vi "After Launch Init.vi"(8 "error in (no error)":errorcluster, 11 "CS++Fgen in":refnum<class "CS++Fgen.lvclass">) -> (0 "error out":errorcluster, 3 "CS++Fgen out":refnum<class "CS++Fgen.lvclass">)   [LabVIEW 2013, in "CS++Fgen.lvlib" / "CS++Fgen.lvclass"]
doc: "Use <b>Pre Launch init.vi</b> method for sanity checks that are supposed to prevent the actor from launching if they fail. Use <B>this</B> method instead to initialize this actor when it has been activated. A corresponding high priority message will become dispatched before the <B>Actor Core.vi</b> is called.\n\n<b>Derived classed should call the parent methode first</b> and their own initialization code after.\n\nRefer also to the ongoing discussion at https://decibel.ni.com/content/message/57394#57394."
uses:
  CS++Fgen.lvclass
  Core/Classes/CS++ProcessVariables/ProcessVariable/PV.lvclass
  Core/Classes/CS++ProcessVariables/SVConnection/SVConnection.lvclass
  CS++Fgen.lvclass/CS++Fgen.ctl
  Core/Classes/CS++ProcessVariables/ProcessVariable/PV.lvclass/PV.ctl
  Core/Classes/CS++ProcessVariables/PVConnection/PVConnection.lvclass/PVConnection.ctl
  Core/Actors/CS++DeviceActor/CS++DeviceActor.lvclass
  Core/Actors/CS++DeviceActor/CS++DeviceActor.lvclass/CS++DeviceActor.ctl
  <vilib>/ActorFramework/Actor/Actor.lvclass/Actor.ctl
  <vilib>/ActorFramework/Message Enqueuer/Message Enqueuer.lvclass/Message Enqueuer.ctl
  CS++DCPwr Messages/Measure [MSR] Msg/Measure [MSR] Msg.lvclass/Measure [MSR] Msg.ctl
  CS++DCPwr Messages/Measure [MSR] Msg/Write channel name.vi
  CS++DCPwr Messages/Measure [MSR] Msg/Write measurement type.vi
  Core/Classes/CS++ProcessVariables/ProcessVariable/Write PV URL.vi
  Core/Classes/CS++ProcessVariables/ProcessVariable/Write Data.vi
  Core/Classes/CS++ProcessVariables/ProcessVariable/Write Error.vi
  Core/Classes/CS++ProcessVariables/ProcessVariable/Write Quality.vi
  Core/Classes/CS++ProcessVariables/ProcessVariable/Write status.vi
  Core/Classes/CS++ProcessVariables/ProcessVariable/Write Timestamp.vi
  Core/Classes/CS++ProcessVariables/PVConnection/Write PV URL.vi
  <vilib>/ActorFramework/Message Enqueuer/Init from Existing Queue.vi
  <vilib>/ActorFramework/Message Enqueuer/Message Enqueuer.lvclass
  CS++DCPwr Messages/Measure [MSR] Msg/Measure [MSR] Msg.lvclass
  <vilib>/ActorFramework/Actor/Actor.lvclass
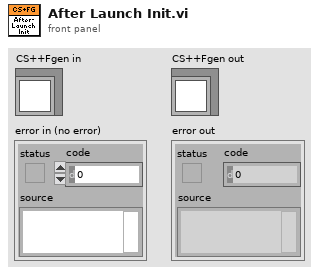
[diagram p1: front panel]
types:
  T1 = cluster{"Write Access":enum8{"Allowed", "Required", "None"}, "Read Access":enum8{"Allowed", "Required", "None"}}
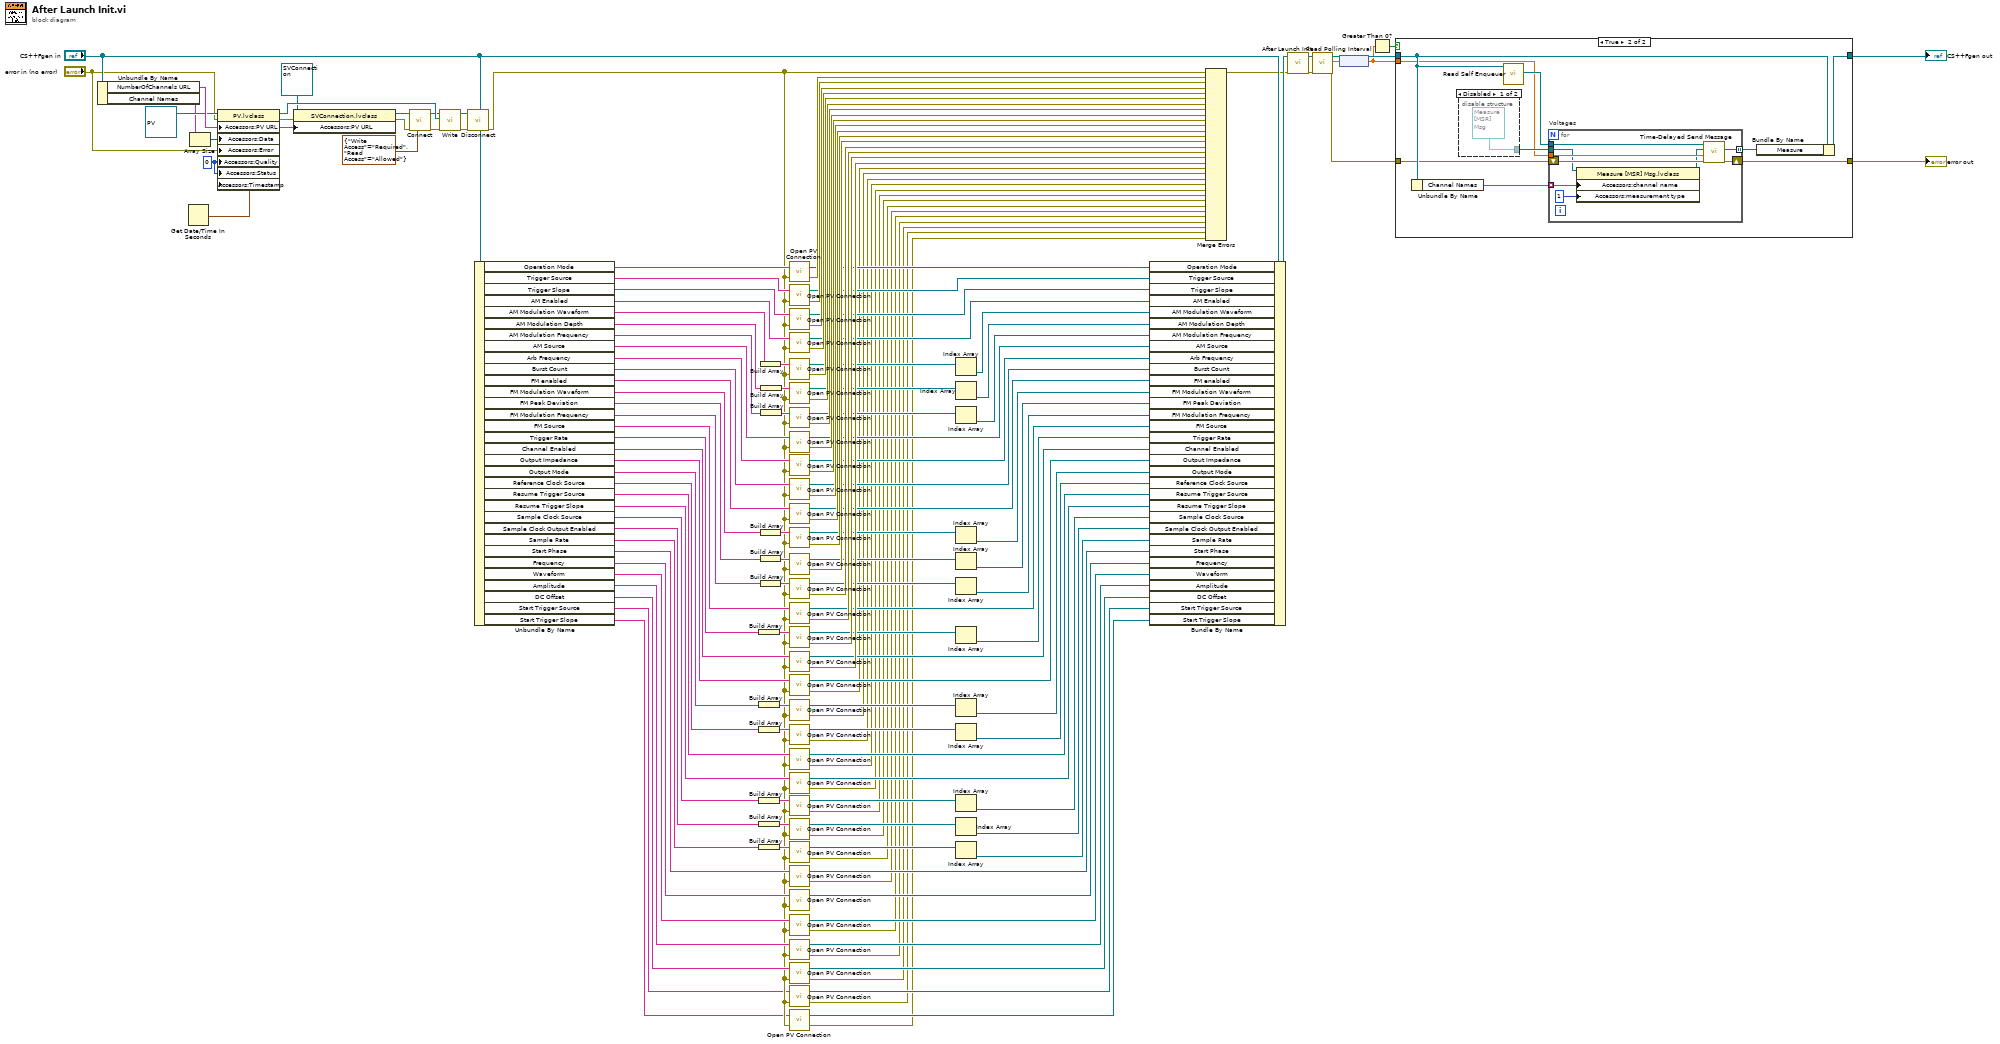
[diagram p0: block diagram]
diagram:
  w137 = 0 ("Quality")
  n1 = Unbundle By Name("CS++Fgen in") -> ("NumberOfChannels URL"=w141:string, "Channel Names"=w134:string[])
  n2 = Get Date/Time In Seconds() -> (seconds since 1Jan1904=w138:timestamp)
  n3 = Array Size(array=w134) -> (size(s)=w136:i32)
  n4 = property class="PV.lvclass"(reference=refnum<class "PV.lvclass"> refnum ("CS++ProcessVariables.lvlib:PV.lvclass"), error in="error in (no error)", "Accessors:PV URL"=w141, "Accessors:Data"=w136, "Accessors:Error"="error in (no error)", "Accessors:Quality"=w137, "Accessors:Status"=w137, "Accessors:Timestamp"=w138) -> (reference out=w147:refnum<class "PV.lvclass">, error out=w142:errorcluster)
  n5 = property class="SVConnection.lvclass"(reference=refnum<class "SVConnection.lvclass"> refnum ("CS++ProcessVariables.lvlib:SVConnection.lvclass"), error in=w142, "Accessors:PV URL"=w141) -> (reference out=w140:refnum<class "SVConnection.lvclass">, error out=w143:errorcluster)
  n6 = call-dynamic "Connect.vi"("Access"=T1 {"Write Access"=enum."Required", "Read Access"=enum."Allowed"}, "error in (no error)"=w143, "PVConnection in"=w140) -> ("error out"=w146:errorcluster, "PVConnection out"=w145:refnum<class "SVConnection.lvclass">)  [unwired: 7 in]
  n7 = call-dynamic "Write.vi"("error in (no error)"=w146, "PV"=w147, "PVConnection in"=w145) -> ("error out"=w149:errorcluster, "PVConnection out"=w148:refnum<class "SVConnection.lvclass">)  [unwired: 7 in]
  n8 = call-dynamic "Disconnect.vi"("error in (no error)"=w149, "PVConnection in"=w148) -> ("error out"=w7:errorcluster)  [unwired: 8 in, 1 out]
  n9 = Unbundle By Name("CS++Fgen in") -> ("Operation Mode"=w133:string[], "Trigger Source"=w101:string[], "Trigger Slope"=w100:string[], "AM Enabled"=w97:string[], "AM Modulation Waveform"=w95:string, "AM Modulation Depth"=w91:string, "AM Modulation Frequency"=w90:string, "AM Source"=w83:string[], "Arb Frequency"=w81:string[], "Burst Count"=w79:string[], "FM enabled"=w77:string[], "FM Modulation Waveform"=w75:string, "FM Peak Deviation"=w71:string, "FM Modulation Frequency"=w70:string, "FM Source"=w69:string[], "Trigger Rate"=w61:string, "Channel Enabled"=w57:string[], "Output Impedance"=w55:string[], "Output Mode"=w50:string, "Reference Clock Source"=w45:string, "Resume Trigger Source"=w42:string[], "Resume Trigger Slope"=w41:string[], "Sample Clock Source"=w34:string, "Sample Clock Output Enabled"=w29:string, "Sample Rate"=w24:string, "Start Phase"=w21:string[], "Frequency"=w20:string[], "Waveform"=w19:string[], "Amplitude"=w18:string[], "DC Offset"=w17:string[], "Start Trigger Source"=w6:string[], "Start Trigger Slope"=w5:string[])
  n10 = Build Array(w61) -> (w60:string[])
  n11 = Build Array(w50) -> (w51:string[])
  n12 = Build Array(w45) -> (w47:string[])
  n13 = Build Array(w34) -> (w35:string[])
  n14 = Build Array(w29) -> (w31:string[])
  n15 = Build Array(w24) -> (w25:string[])
  n16 = Build Array(w95) -> (w94:string[])
  n17 = Build Array(w75) -> (w74:string[])
  n18 = Build Array(w71) -> (w68:string[])
  n19 = Build Array(w70) -> (w67:string[])
  n20 = Build Array(w91) -> (w93:string[])
  n21 = Build Array(w90) -> (w92:string[])
  n22 = call "Open PV Connection.vi"("Error In"=w7, "URLs"=w133) -> ("Error Out"=w132:errorcluster, "PV Connections"=w113:refnum<class "SVConnection.lvclass">[])
  n23 = call "Open PV Connection.vi"("Error In"=w7, "URLs"=w101) -> ("Error Out"=w131:errorcluster, "PV Connections"=w99:refnum<class "SVConnection.lvclass">[])
  n24 = call "Open PV Connection.vi"("Error In"=w7, "URLs"=w100) -> ("Error Out"=w130:errorcluster, "PV Connections"=w98:refnum<class "SVConnection.lvclass">[])
  n25 = call "Open PV Connection.vi"("Error In"=w7, "URLs"=w97) -> ("Error Out"=w129:errorcluster, "PV Connections"=w96:refnum<class "SVConnection.lvclass">[])
  n26 = call "Open PV Connection.vi"("Error In"=w7, "URLs"=w94) -> ("Error Out"=w128:errorcluster, "PV Connections"=w89:refnum<class "SVConnection.lvclass">[])
  n27 = call "Open PV Connection.vi"("Error In"=w7, "URLs"=w93) -> ("Error Out"=w127:errorcluster, "PV Connections"=w87:refnum<class "SVConnection.lvclass">[])
  n28 = call "Open PV Connection.vi"("Error In"=w7, "URLs"=w92) -> ("Error Out"=w126:errorcluster, "PV Connections"=w84:refnum<class "SVConnection.lvclass">[])
  n29 = call "Open PV Connection.vi"("Error In"=w7, "URLs"=w83) -> ("Error Out"=w125:errorcluster, "PV Connections"=w82:refnum<class "SVConnection.lvclass">[])
  n30 = call "Open PV Connection.vi"("Error In"=w7, "URLs"=w81) -> ("Error Out"=w124:errorcluster, "PV Connections"=w80:refnum<class "SVConnection.lvclass">[])
  n31 = call "Open PV Connection.vi"("Error In"=w7, "URLs"=w79) -> ("Error Out"=w123:errorcluster, "PV Connections"=w78:refnum<class "SVConnection.lvclass">[])
  n32 = call "Open PV Connection.vi"("Error In"=w7, "URLs"=w77) -> ("Error Out"=w122:errorcluster, "PV Connections"=w76:refnum<class "SVConnection.lvclass">[])
  n33 = call "Open PV Connection.vi"("Error In"=w7, "URLs"=w74) -> ("Error Out"=w121:errorcluster, "PV Connections"=w73:refnum<class "SVConnection.lvclass">[])
  n34 = call "Open PV Connection.vi"("Error In"=w7, "URLs"=w68) -> ("Error Out"=w120:errorcluster, "PV Connections"=w66:refnum<class "SVConnection.lvclass">[])
  n35 = call "Open PV Connection.vi"("Error In"=w7, "URLs"=w67) -> ("Error Out"=w119:errorcluster, "PV Connections"=w65:refnum<class "SVConnection.lvclass">[])
  n36 = call "Open PV Connection.vi"("Error In"=w7, "URLs"=w69) -> ("Error Out"=w118:errorcluster, "PV Connections"=w62:refnum<class "SVConnection.lvclass">[])
  n37 = call "Open PV Connection.vi"("Error In"=w7, "URLs"=w60) -> ("Error Out"=w117:errorcluster, "PV Connections"=w59:refnum<class "SVConnection.lvclass">[])
  n38 = call "Open PV Connection.vi"("Error In"=w7, "URLs"=w57) -> ("Error Out"=w116:errorcluster, "PV Connections"=w56:refnum<class "SVConnection.lvclass">[])
  n39 = call "Open PV Connection.vi"("Error In"=w7, "URLs"=w55) -> ("Error Out"=w53:errorcluster, "PV Connections"=w54:refnum<class "SVConnection.lvclass">[])
  n40 = call "Open PV Connection.vi"("Error In"=w7, "URLs"=w51) -> ("Error Out"=w48:errorcluster, "PV Connections"=w52:refnum<class "SVConnection.lvclass">[])
  n41 = call "Open PV Connection.vi"("Error In"=w7, "URLs"=w47) -> ("Error Out"=w43:errorcluster, "PV Connections"=w46:refnum<class "SVConnection.lvclass">[])
  n42 = call "Open PV Connection.vi"("Error In"=w7, "URLs"=w42) -> ("Error Out"=w38:errorcluster, "PV Connections"=w40:refnum<class "SVConnection.lvclass">[])
  n43 = call "Open PV Connection.vi"("Error In"=w7, "URLs"=w41) -> ("Error Out"=w37:errorcluster, "PV Connections"=w39:refnum<class "SVConnection.lvclass">[])
  n44 = call "Open PV Connection.vi"("Error In"=w7, "URLs"=w35) -> ("Error Out"=w32:errorcluster, "PV Connections"=w36:refnum<class "SVConnection.lvclass">[])
  n45 = call "Open PV Connection.vi"("Error In"=w7, "URLs"=w31) -> ("Error Out"=w27:errorcluster, "PV Connections"=w30:refnum<class "SVConnection.lvclass">[])
  n46 = call "Open PV Connection.vi"("Error In"=w7, "URLs"=w25) -> ("Error Out"=w22:errorcluster, "PV Connections"=w26:refnum<class "SVConnection.lvclass">[])
  n47 = call "Open PV Connection.vi"("Error In"=w7, "URLs"=w21) -> ("Error Out"=w11:errorcluster, "PV Connections"=w16:refnum<class "SVConnection.lvclass">[])
  n48 = call "Open PV Connection.vi"("Error In"=w7, "URLs"=w20) -> ("PV Connections"=w15:refnum<class "SVConnection.lvclass">[])  [unwired: 1 out]
  n49 = call "Open PV Connection.vi"("Error In"=w7, "URLs"=w19) -> ("Error Out"=w10:errorcluster, "PV Connections"=w14:refnum<class "SVConnection.lvclass">[])
  n50 = call "Open PV Connection.vi"("Error In"=w7, "URLs"=w18) -> ("Error Out"=w9:errorcluster, "PV Connections"=w13:refnum<class "SVConnection.lvclass">[])
  n51 = call "Open PV Connection.vi"("Error In"=w7, "URLs"=w17) -> ("Error Out"=w8:errorcluster, "PV Connections"=w12:refnum<class "SVConnection.lvclass">[])
  n52 = call "Open PV Connection.vi"("Error In"=w7, "URLs"=w6) -> ("Error Out"=w2:errorcluster, "PV Connections"=w4:refnum<class "SVConnection.lvclass">[])
  n53 = call "Open PV Connection.vi"("Error In"=w7, "URLs"=w5) -> ("Error Out"=w1:errorcluster, "PV Connections"=w3:refnum<class "SVConnection.lvclass">[])
  n54 = Index Array(array=w89) -> (element=w88:refnum<class "SVConnection.lvclass">)  [unwired: 1 in]
  n55 = Index Array(array=w87) -> (element=w86:refnum<class "SVConnection.lvclass">)  [unwired: 1 in]
  n56 = Index Array(array=w84) -> (element=w85:refnum<class "SVConnection.lvclass">)  [unwired: 1 in]
  n57 = Index Array(array=w73) -> (element=w72:refnum<class "SVConnection.lvclass">)  [unwired: 1 in]
  n58 = Index Array(array=w66) -> (element=w64:refnum<class "SVConnection.lvclass">)  [unwired: 1 in]
  n59 = Index Array(array=w65) -> (element=w63:refnum<class "SVConnection.lvclass">)  [unwired: 1 in]
  n60 = Index Array(array=w59) -> (element=w58:refnum<class "SVConnection.lvclass">)  [unwired: 1 in]
  n61 = Index Array(array=w52) -> (element=w49:refnum<class "SVConnection.lvclass">)  [unwired: 1 in]
  n62 = Index Array(array=w46) -> (element=w44:refnum<class "SVConnection.lvclass">)  [unwired: 1 in]
  n63 = Index Array(array=w36) -> (element=w33:refnum<class "SVConnection.lvclass">)  [unwired: 1 in]
  n64 = Index Array(array=w30) -> (element=w28:refnum<class "SVConnection.lvclass">)  [unwired: 1 in]
  n65 = Index Array(array=w26) -> (element=w23:refnum<class "SVConnection.lvclass">)  [unwired: 1 in]
  n66 = Bundle By Name(cluster="CS++Fgen in", "Operation Mode"=w113, "Trigger Source"=w99, "Trigger Slope"=w98, "AM Enabled"=w96, "AM Modulation Waveform"=w88, "AM Modulation Depth"=w86, "AM Modulation Frequency"=w85, "AM Source"=w82, "Arb Frequency"=w80, "Burst Count"=w78, "FM enabled"=w76, "FM Modulation Waveform"=w72, "FM Peak Deviation"=w64, "FM Modulation Frequency"=w63, "FM Source"=w62, "Trigger Rate"=w58, "Channel Enabled"=w56, "Output Impedance"=w54, "Output Mode"=w49, "Reference Clock Source"=w44, "Resume Trigger Source"=w40, "Resume Trigger Slope"=w39, "Sample Clock Source"=w33, "Sample Clock Output Enabled"=w28, "Sample Rate"=w23, "Start Phase"=w16, "Frequency"=w15, "Waveform"=w14, "Amplitude"=w13, "DC Offset"=w12, "Start Trigger Source"=w4, "Start Trigger Slope"=w3) -> (w114:refnum<class "CS++Fgen.lvclass">)
  n67 = Merge Errors(w7, w132, w131, w130, w129, w128, w127, w126, w125, w124, w123, w122, w121, w120, w119, w118, w117, w116, w53, w48, w43, w38, w37, w32, w27, w22, w11, w10, w9, w8, w2, w1) -> (w102:errorcluster)
  n68 = call-parent "After Launch Init.vi"("error in (no error)"=w102, "CS++DeviceActor in"=w114) -> ("error out"=w105:errorcluster, "CS++DeviceActor out"=w106:refnum<class "CS++Fgen.lvclass">)  [unwired: 8 in]
  n69 = call "Read Polling Interval.vi"("error in (no error)"=w105, "CS++DeviceActor in"=w106) -> ("error out"=w110:errorcluster, "Polling Interval"=w109:dbl[unit], "CS++DeviceActor out"=w111:refnum<class "CS++Fgen.lvclass">)  [unwired: 7 in]
  n70 = node(w109) -> (w108:dbl)
  n71 = Greater Than 0?(x=w108) -> (x > 0?=w107:bool)
  n72 = case shown="True" w107 {
    tunnel: [w151 w160] -> w104
    tunnel: [w150 w152] -> w103
    tunnel: w111 -> [w151 w159]
    tunnel: w110 -> [w150 w156]
    tunnel: w108 -> [_ w155]
    frame False {
    }
    frame True {
      n73 = Unbundle By Name(w159) -> ("Channel Names"=w154:string[])
      n74 = disable-structure shown="Disabled" {
        disable-tunnel: [refnum<class "Measure [MSR] Msg.lvclass"> refnum ("CS++DCPwr.lvlib:Measure [MSR] Msg.lvclass") _] -> w158
        frame Disabled {
        }
        frame Enabled {
        }
      }
      n75 = call <vilib>:"Read Self Enqueuer.vi"("Actor"=w159) -> ("Self Enqueuer"=w157:refnum<class "Message Enqueuer.lvclass">)  [unwired: 10 in]
      n76 = for "Voltages" {
        tunnel: w157 -> [w169]
        tunnel: w155 -> [w167]
        tunnel: [w166] -> w153 mode=indexing
        tunnel: w158 -> [w162]
        shift-right: [w170] -> w152
        shift-left: w156 -> [w168]
        tunnel: w154 -> [w165] mode=indexing
        n77 = property class="Measure [MSR] Msg.lvclass"(reference=w162, "Accessors:channel name"=w165, "Accessors:measurement type"=1 ("measurement type (voltage)")) -> (reference out=w163:refnum<class "Measure [MSR] Msg.lvclass">)  [unwired: 1 in, 1 out]
        n78 = call <vilib>:"Time-Delayed Send Message.vi"("error in (no error)"=w168, "Milliseconds To Wait"=w167, "Message"=w163, "Message Enqueuer"=w169) -> ("error out"=w170:errorcluster, "Delivery Notifier"=w166:refnum<notifier>)  [unwired: 6 in]
      }
      n79 = Bundle By Name(cluster=w159, "Measure"=w153) -> (w160:refnum<class "CS++Fgen.lvclass">)
    }
  }
  "error out" <- w103
  "CS++Fgen out" <- w104
